vi "Panel Build GUI Control.vi"(8 "error in (no error)":errorcluster, 11 "Panel Control_Ref in":refnum<class "Panel Controller.lvclass">) -> (0 "error out":errorcluster, 2 "Panel Request Behavior":refnum<class "Panel Behavior.lvclass">, 3 "Panel Control_Ref out":refnum<class "Panel Controller.lvclass">)   [LabVIEW 2015, in "Panel Controller.lvclass"]
uses:
  Panel Controller.lvclass
  _Depences/Panel API/Panel Request/Panle Requeset Behavior/Panel Behavior.lvclass
  GUI/GUI Builder Director/GUI Control Builder Director.lvclass
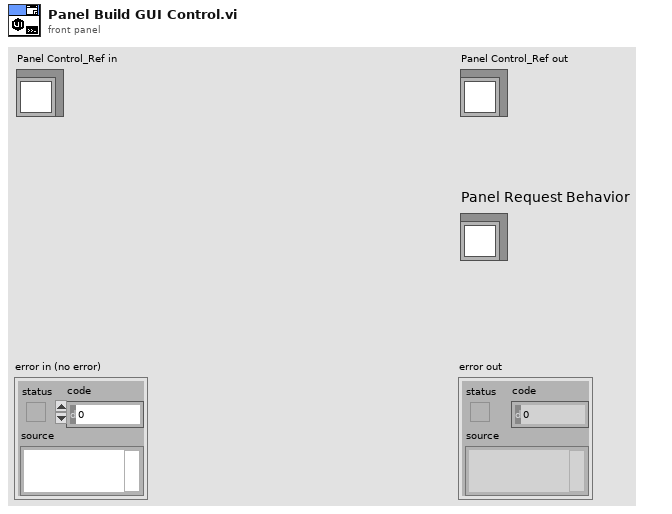
[diagram p1: front panel]
types:
  T1 = typedef "Panel Controller.lvclass/ObjectAttributes.ctl" = cluster{"Sub Panel Ref":refnum<vi>, "Panel_Q":refnum<queue>, "VI Running Refnum":refnum<vi>, "Brower Controller_Q":refnum<class "Message Enqueuer.lvclass">, "GUI Control Builder Director.lvclass":refnum<class "GUI Control Builder Director.lvclass">, "Panel GUI Manager.lvclass":refnum<class "Panel GUI Manager.lvclass">}
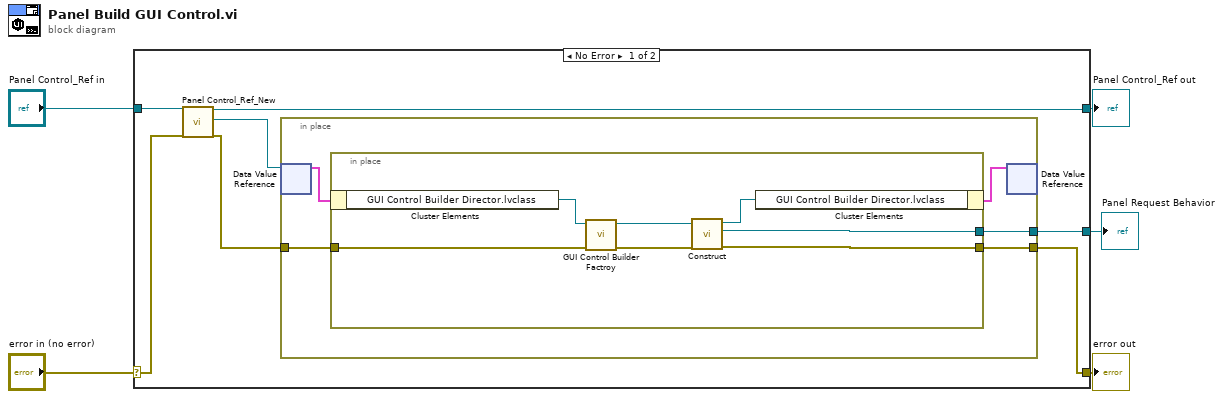
[diagram p0: block diagram]
diagram:
  n1 = case shown="No Error" "error in (no error)" {
    selector: "error in (no error)" -> [w10 w26]
    tunnel: [w7 w26] -> w4
    tunnel: [w6 w25] -> w2
    tunnel: "Panel Control_Ref in" -> [w11 w25]
    tunnel: [w12 _] -> w1
    frame No Error {
      n2 = call "Panel Control_Ref_New.vi"("reference in"=w11, "error in (no error)"=w10) -> ("reference out"=w6:refnum<class "Panel Controller.lvclass">, "DVRRefOut"=w9:refnum<data-value>, "error out"=w8:errorcluster)  [unwired: 14 in, 1 out]
      n3 = in-place {
        in-place-border: [w17] -> w12
        in-place-border: w8 -> [w15]
        in-place-border: [w14] -> w7
        n4 = in-place-dvr #1(w9) -> (w16:T1)  [unwired: 1 out]
        n5 = in-place {
          in-place-border: [w24] -> w17
          in-place-border: w15 -> [w20]
          in-place-border: [w22] -> w14
          n6 = in-place-cluster #2(w16) -> ("GUI Control Builder Director.lvclass"=w21:refnum<class "GUI Control Builder Director.lvclass">)
          n7 = call "GUI Control Builder Factroy.vi"("error in (no error)"=w20, "GUI Control Builder Director in"=w21) -> ("error out"=w18:errorcluster, "GUI Control Builder Director out"=w19:refnum<class "GUI Control Builder Director.lvclass">)  [unwired: 7 in, 1 out]
          n8 = call "Construct.vi"("error in (no error)"=w18, "GUI Control Builder Director in"=w19) -> ("error out"=w22:errorcluster, "Panel Request Behavior"=w24:refnum<class "Panel Behavior.lvclass">, "GUI Control Builder Director out"=w23:refnum<class "GUI Control Builder Director.lvclass">)  [unwired: 7 in]
          n9 = in-place-cluster #2("GUI Control Builder Director.lvclass"=w23) -> (w13:T1)
        }
        n10 = in-place-dvr #1(w13) -> ()  [unwired: 2 out]
      }
    }
    frame Error {
    }
  }
  "error out" <- w4
  "Panel Control_Ref out" <- w2
  "Panel Request Behavior" <- w1
